vi "Create AChange Error.vi"(0 "reference in":refnum<class "Stand.lvclass">, 1 "size (10)":u32, 2 "default value":dbl[](array[numeric]), 11 "error in (no error)":errorcluster) -> (4 "reference out":refnum<class "Stand.lvclass">, 15 "error out":errorcluster)   [LabVIEW 2019, in "Stand.lvclass"]
uses:
  Stand.lvclass
  D:/GIT H4000/H4000/src/Proccess_class/Proccess.lvclass
  Stand.lvclass/Stand.ctl
  Proccess_class/Proccess.lvclass/Proccess.ctl
  Proccess_class/TAGs.ctl
  TypeDef/AlarmType.ctl
  Proccess_class/Proccess.lvclass
  AbruptChange_class/AnalogComparator_class/AbruptChange.lvclass
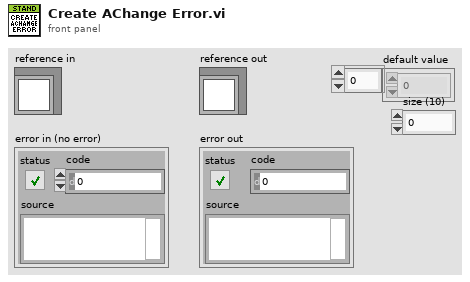
[diagram p1: front panel]
types:
  T1 = typedef "AlarmType.ctl" = enum16{"Normal", "Warning", "Alarm"}
  T2 = typedef "Proccess.lvclass/TAGs.ctl" = cluster{"TAG":string, "PTAG":string, "DESC":string}
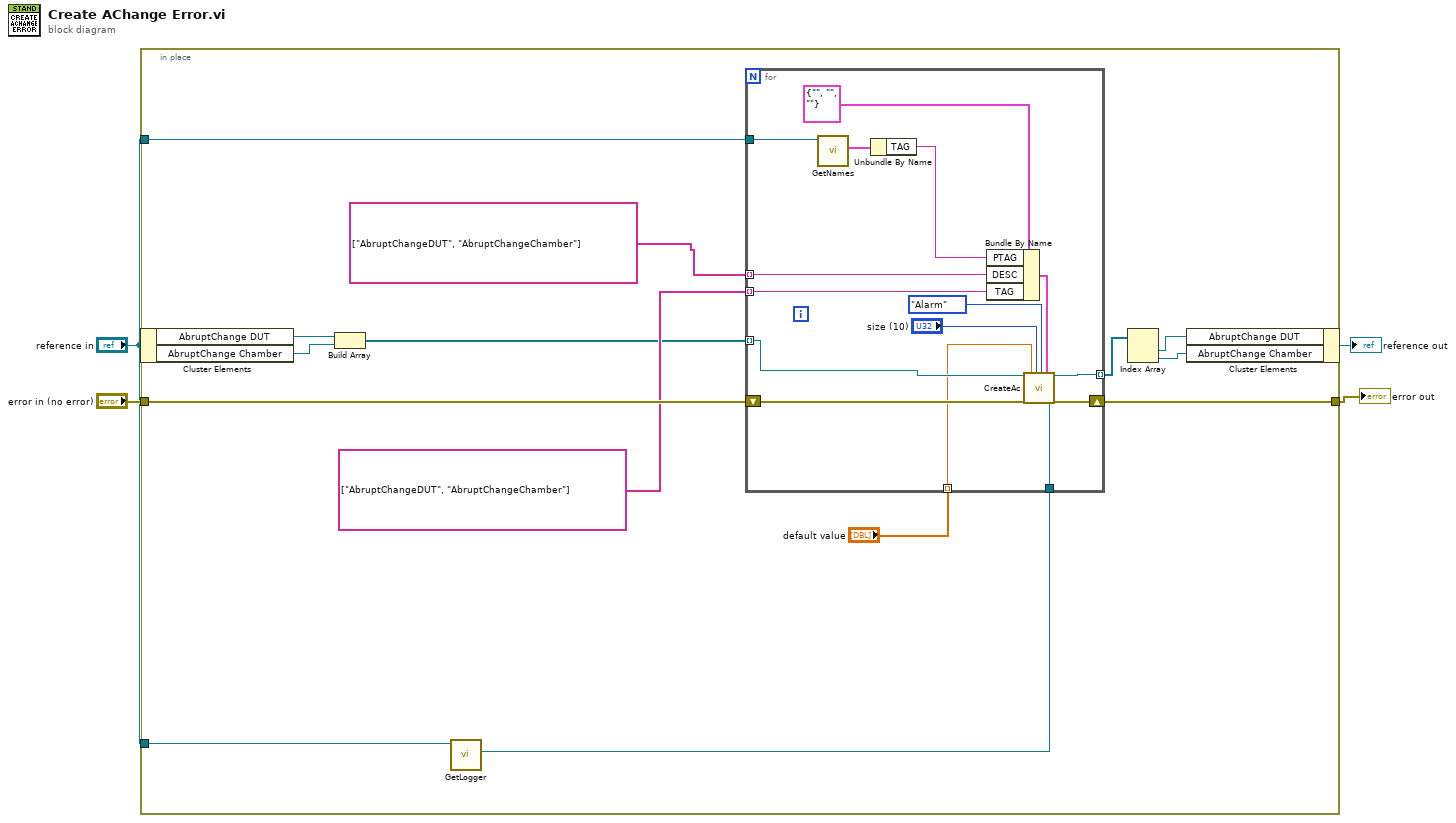
[diagram p0: block diagram]
diagram:
  n1 = in-place {
    in-place-border: "error in (no error)" -> [w18]
    in-place-border: "reference in" -> [w17]
    in-place-border: "reference in" -> [w16]
    in-place-border: [w14] -> w1
    n2 = in-place-cluster #1("reference in") -> ("AbruptChange DUT"=w12:refnum<class "AbruptChange.lvclass">, "AbruptChange Chamber"=w11:refnum<class "AbruptChange.lvclass">)
    n3 = Build Array(w12, w11) -> (w7:refnum<class "AbruptChange.lvclass">[])
    n4 = call "GetLogger.vi"("Proccess in"=w16) -> ("Logger"=w15:refnum<class "Logger.lvclass">)  [unwired: 10 in]
    n5 = for {
      tunnel: [w32] -> w10 mode=indexing
      shift-right: [w31] -> w14
      shift-left: w18 -> [w33]
      tunnel: string[] ["AbruptChangeDUT", "AbruptChangeChamber"] -> [w28] mode=indexing
      tunnel: w17 -> [w25]
      tunnel: w15 -> [w24]
      tunnel: string[] ["AbruptChangeDUT", "AbruptChangeChamber"] -> [w23] mode=indexing
      tunnel: w7 -> [w22] mode=indexing
      tunnel: "default value" -> [w19] mode=indexing
      n6 = call "GetNames.vi"("Proccess in"=w25) -> ("Tags"=w27:T2)  [unwired: 10 in]
      n7 = Unbundle By Name(w27) -> ("TAG"=w26:string)
      n8 = Bundle By Name(cluster=T2 {"TAG"="", "PTAG"="", "DESC"=""} ("Tags"), "PTAG"=w26, "DESC"=w28, "TAG"=w23) -> (w29:T2)
      n9 = call "CreateAc.vi"("Abrupt Change"=w22, "error in (no error)"=w33, "default value"=w19, "size (10)"="size (10)", "AlarmType"=AlarmType."Alarm", "Tags"=w29, "Logger"=w24) -> ("AnalogComparator out"=w32:refnum<class "AbruptChange.lvclass">, "error out"=w31:errorcluster)  [unwired: 11 in]
    }
    n10 = Index Array(array=w10) -> (element #1=w9:refnum<class "AbruptChange.lvclass">, element #2=w8:refnum<class "AbruptChange.lvclass">)  [unwired: 2 in]
    n11 = in-place-cluster #1("AbruptChange DUT"=w9, "AbruptChange Chamber"=w8) -> (→"reference out":refnum<class "Stand.lvclass">)
  }
  "error out" <- w1
